vi "Add Hx to the orginal value.vi"(0 "A Out":u32, 1 "H0 In":u32, 2 "H1 In":u32, 5 "B Out":u32, 7 "C Out":u32, 9 "D Out":u32, 11 "E Out":u32, 12 "H2 In":u32, 13 "H3 In":u32, 14 "H4 In":u32) -> (4 "H0":u32 format="%x", 6 "H1":u32 format="%x", 8 "H2":u32 format="%x", 10 "H3":u32 format="%x", 15 "H4":u32 format="%x")   [LabVIEW 2014]
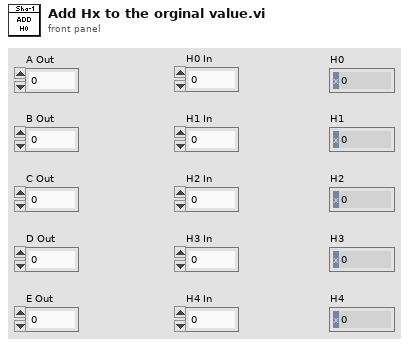
[diagram p1: front panel]
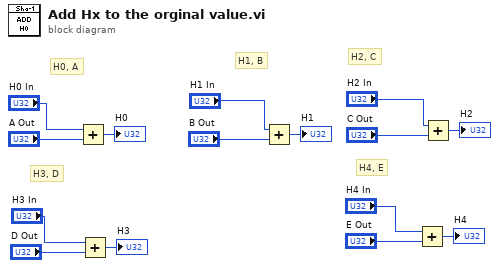
[diagram p0: block diagram]
diagram:
  # "H0, A"
  # "H4, E"
  # "H3, D"
  # "H2, C"
  # "H1, B"
  n1 = Add(x="H0 In", y="A Out") -> (x+y=→"H0":u32)
  n2 = Add(x="H3 In", y="D Out") -> (x+y=→"H3":u32)
  n3 = Add(x="H1 In", y="B Out") -> (x+y=→"H1":u32)
  n4 = Add(x="H4 In", y="E Out") -> (x+y=→"H4":u32)
  n5 = Add(x="H2 In", y="C Out") -> (x+y=→"H2":u32)
